vi "DI DAQ.vi"(11 "Queue ref":T1) -> ()   [LabVIEW 2022 SP3]
uses:
  Controls/All Queue.ctl
  Controls/DAQ case.ctl
  Controls/UI Data.ctl
  Controls/All Loop Status.ctl
  <vilib>/DAQmx/read.llb/DAQmx Read (Digital 1D Wfm NChan NSamp).vi
  Create Task/DI Create Task.vi
  <vilib>/DAQmx/configure/timing.llb/DAQmx Timing (Sample Clock).vi
  <vilib>/DAQmx/configure/trigger.llb/DAQmx Start Trigger (Time).vi
  Sub VI's/Global 1.vi
  <vilib>/DAQmx/miscellaneous.llb/DAQmx Fill In Error Info.vi
panel:
  # "TC channel list"
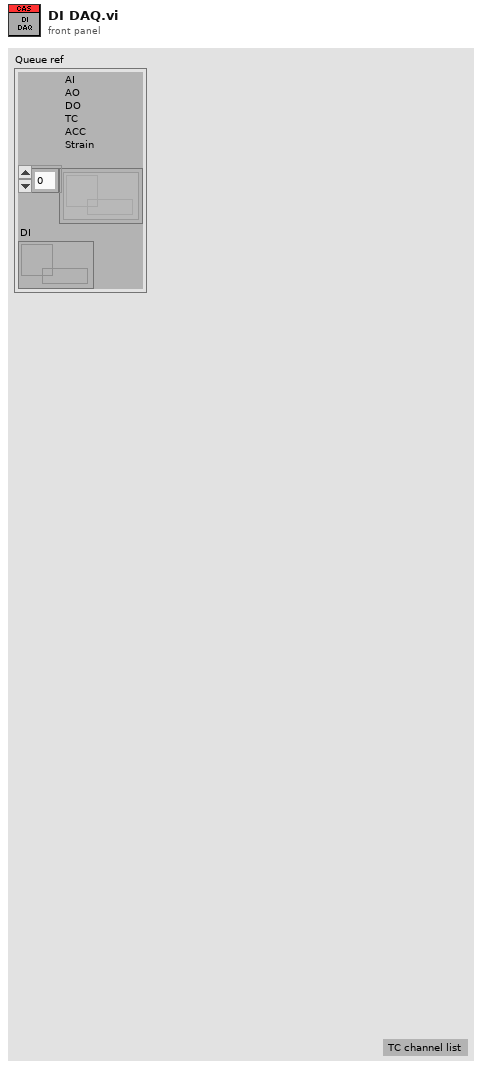
[diagram p1: front panel]
types:
  T1 = typedef "All Queue.ctl" = cluster{"AI\nAO\nDO\nTC\nACC\nStrain":refnum<queue>[], "DI":refnum<queue>}
  T2 = cluster{"in progress?":bool, "Queue ref":T1, "Start DAQ":refnum<notifier>, "UI Data":refnum<notifier>, "task out":refnum<k21>, "AI Ref":refnum<queue>, "SPC":i32}
  T3 = typedef "DAQ case.ctl" = enum16{"Initailise", "Create Task", "Polevent", "Acquire", "Stop DAQ", "Error", "Exit"}
  T4 = typedef "All Loop Status.ctl" = enum16{"AI", "AO", "DI", "DO", "TC", "Strain", "ACC", "RT", "Log"}
  T5 = enum16{"Init", "Read 'All'", "Read 'n'", "Read '1'", "Write '1'", "Write 'n'", "Write 'All'"}
  T6 = typedef "All Notifer.ctl" = cluster{"UI Data":refnum<notifier>, "Start DAQ":refnum<notifier>, "Start Log":refnum<notifier>}
  T7 = cluster{"Analog input":bool, "Analog Output":bool, "Digital input":bool, "Digital output":bool, "Thermocouple":bool, "Strain Gauge":bool, "Accelerometer":bool}
  T8 = typedef "Config.ctl" = cluster{"AO config":cluster{"Channel_Name":string, "Channel_Number":string, "Default_Value":dbl, "Units":string}[], "AI config":cluster{"Channel_Name":string, "Channel_Number":string, "Pre_Scale_min":dbl, "Pre_Scale_max":dbl, "Sensor_min":dbl, "Sensor_max":dbl, "Units":string}[], "DI config":cluster{"Channel_Name":string, "Channel_Number":string, "Default_Value":bool, "DI invert?":bool}[], "DO config":cluster{"Channel_Name":string, "Channel_Number":string, "Default_Value":bool, "DO invert?":bool}[], "TC config":cluster{"Channel_Name":string, "Channel_Number":string, "Pre_Scale_min":dbl, "Pre_Scale_max":dbl, "units":i32, " type":i32}[], "ACC config":cluster{"Channel_Name":string, "Channel_Number":string, "Pre_Scale_min":dbl, "Pre_Scale_max":dbl, "Terminal configuration":i32, "Sensitivity":dbl, "Sensitivity units":i32}[], "SG config":cluster{"Channel_Name":string, "Channel_Number":string, "Pre_Scale_min":dbl, "Pre_Scale_max":dbl}[], "Strain Gauge Settings":cluster{"poisson ratio":dbl, "nominal gage resistance":dbl, "gage factor":dbl}, "bridge information":cluster{"strain configuration":i32, "lead wire resistance":dbl, "initial bridge voltage":dbl, "voltage excitation source":i32, "voltage excitation value":dbl}, "Sample Rate":cluster{"AI Sample Rate":dbl, "AO Sample Rate":dbl, "DI Sample Rate":dbl, "TC Sample Rate":dbl, "DO Sample Rate":dbl, "SG Sample Rate":dbl, "ACC Sample Rate":dbl}}
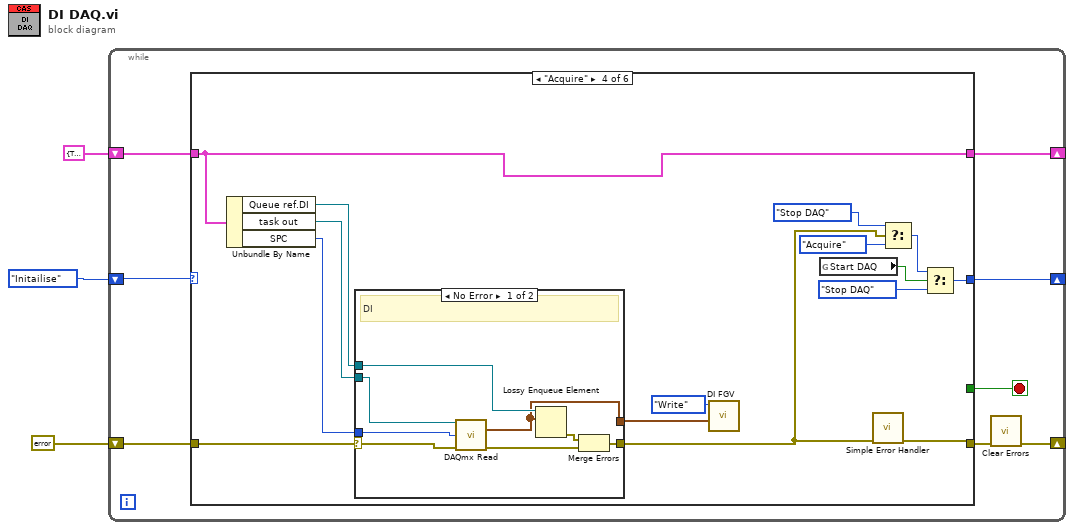
[diagram p0: block diagram]
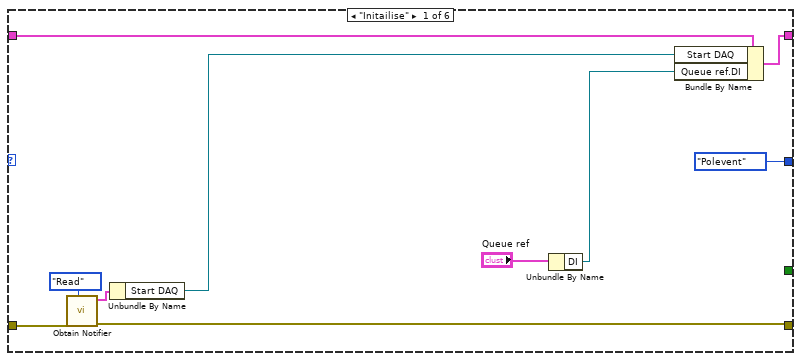
[diagram p2: hidden frame]
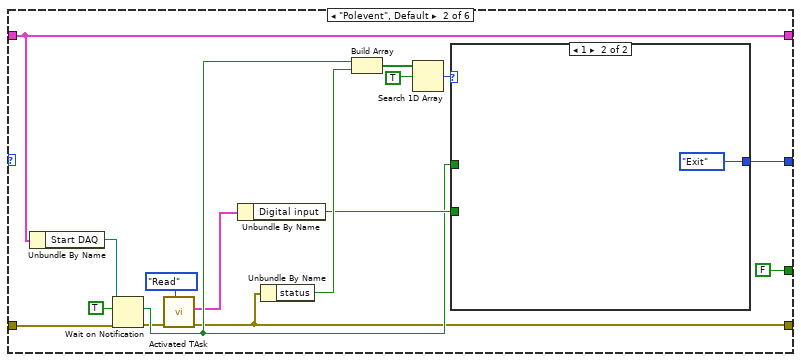
[diagram p3: hidden frame]
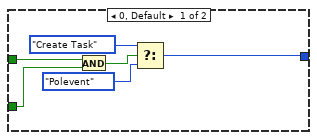
[diagram p4: hidden frame]
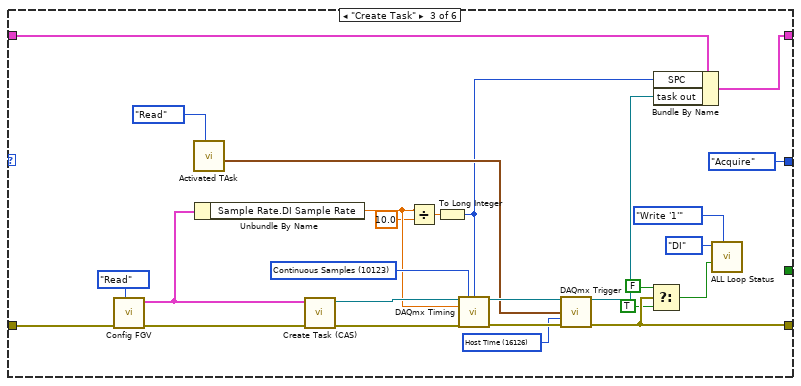
[diagram p5: hidden frame]
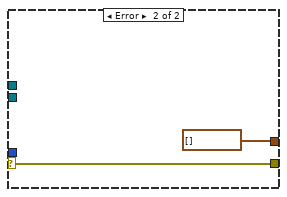
[diagram p6: hidden frame]
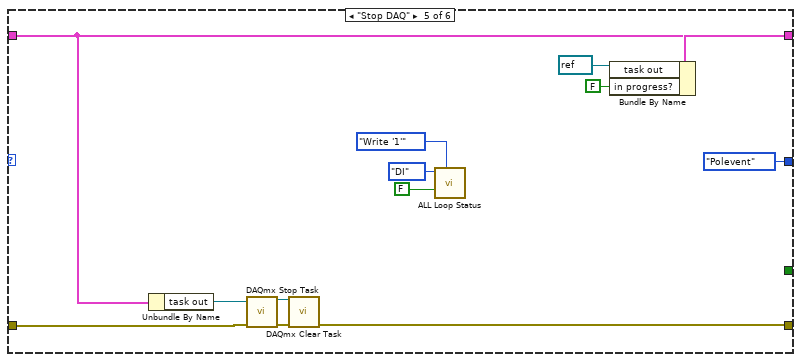
[diagram p7: hidden frame]
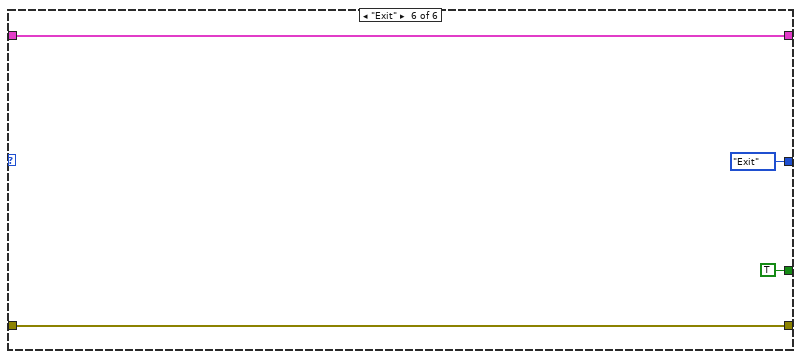
[diagram p8: hidden frame]
diagram:
  n1 = while {
    shift-right: [w4] -> _
    shift-left: errorcluster {"status"=FALSE, "code"=0, "source"=""} ("error out") -> [w10]
    shift-right: [w8] -> _
    shift-left: T2 {"in progress?"=TRUE, "Queue ref"={"AI\nAO\nDO\nTC\nACC\nStrain"=[], "DI"=refnum}, "Start DAQ"=refnum, "UI Data"=refnum, "task out"="", "AI Ref"=refnum, "SPC"=0} -> [w9]
    shift-right: [w7] -> _
    shift-left: DAQ_case."Initailise" -> [w6]
    stop <- w11 stop-if-true
    n2 = case shown="\"Acquire\"" w6 {
      tunnel: [_ FALSE _ _ _ TRUE] -> w11
      tunnel: w10 -> [w20 w25 w67 w78 w100 w112]
      tunnel: [w19 w23 w52 w72 w101 w112] -> w5
      tunnel: w9 -> [w17 w35 w69 w79 w105 w111]
      tunnel: [w15 w35 w68 w79 w106 w111] -> w8
      tunnel: [DAQ_case."Polevent" w36 DAQ_case."Acquire" w80 DAQ_case."Polevent" DAQ_case."Exit"] -> w7
      frame "Initailise" {
        n3 = call "Obtain Notifier.vi"("Case"=enum16{"Obtain", "Read"}."Read", "error in (no error)"=w20) -> ("error out"=w19:errorcluster, "notifiers out"=w18:T6)  [unwired: 8 in]
        n4 = Unbundle By Name(w18) -> ("Start DAQ"=w16:refnum<notifier>)
        n5 = Unbundle By Name("Queue ref") -> ("DI"=w12:refnum<queue>)
        n6 = Bundle By Name(cluster=w17, "Start DAQ"=w16, "Queue ref.DI"=w12) -> (w15:T2)
      }
      frame "Polevent", Default {
        n7 = Unbundle By Name(w35) -> ("Start DAQ"=w34:refnum<notifier>)
        n8 = Wait on Notification(notifier=w34, ignore previous (F)=TRUE, error in (no error)=w25) -> (notification=w26:bool, error out=w24:errorcluster)  [unwired: 1 in, 2 out]
        n9 = call "Activated TAsk.vi"("Enum"=enum16{"Read", "Write"}."Read", "error in (no error)"=w24) -> ("error out"=w23:errorcluster, "Activate Task 2"=w22:T7)  [unwired: 7 in, 1 out]
        n10 = Unbundle By Name(w22) -> ("Digital input"=w27:bool)
        n11 = Unbundle By Name(w23) -> ("status"=w33:bool)
        n12 = Build Array(w26, w33) -> (w31:bool[])
        n13 = Search 1D Array(1D array=w31, element=TRUE) -> (index of element=w29:i32)  [unwired: 1 in]
        n14 = case shown="1" w29 {
          tunnel: [w42 DAQ_case."Exit"] -> w36
          tunnel: w27 -> [w39 _]
          tunnel: w26 -> [w38 _]
          frame 0, Default {
            n15 = And(x=w38, y=w39) -> (x .and. y?=w40:bool)
            n16 = Select(t=DAQ_case."Create Task", s=w40, f=DAQ_case."Polevent") -> (s? t:f=w42:T3)
          }
          frame 1 {
          }
        }
      }
      frame "Create Task" {
        w57 = 16126 items=["Host Time"=16126, "I/O Device Time"=16127] ("timescale")
        w59 = 10123 items=["Finite Samples"=10178, "Continuous Samples"=10123, "Hardware Timed Single Point"=12522] ("sample mode")
        n17 = call "Config FGV.vi"("Enum"=enum16{"Read", "Write"}."Read", "error in (no error)"=w67) -> ("error out"=w64:errorcluster, "Data"=w49:T8)  [unwired: 8 in]
        n18 = call "Activated TAsk.vi"("Enum"=enum16{"Read", "Write"}."Read") -> ("Start Time"=w58:timestamp)  [unwired: 8 in, 2 out]
        n19 = Unbundle By Name(w49) -> ("Sample Rate.DI Sample Rate"=w48:dbl)
        n20 = call-poly "Create Task (CAS).vi"("error in"=w64, "Config"=w49) -> ("error out"=w61:errorcluster, "DI Task"=w63:refnum<k21>)  [unwired: 7 in, 1 out]
        n21 = Divide(x=w48, y=10.0) -> (x/y=w46:dbl)
        n22 = To Long Integer(number=w46) -> (32bit integer=w45:i32)
        n23 = call-poly <vilib>:"DAQmx Timing.vi"("task/channels in"=w63, "sample mode"=w59, "samples per channel"=w45, "rate"=w48, "error in"=w61) -> ("task out"=w62:refnum<k21>, "error out"=w60:errorcluster)  [unwired: 9 in]
        n24 = call-poly <vilib>:"DAQmx Trigger.vi"("task/channels in"=w62, "when"=w58, "timescale"=w57, "error in"=w60) -> ("task out"=w56:refnum<k21>, "error out"=w52:errorcluster)  [unwired: 10 in]
        n25 = Select(t=FALSE, s=w52, f=TRUE) -> (s? t:f=w53:bool)
        n26 = Bundle By Name(cluster=w69, "SPC"=w45, "task out"=w56) -> (w68:T2)
        n27 = call "ALL Loop Status.vi"("Option"=T5."Write '1'", "Status"=w53, "Loop"=All_Loop_Status."DI") -> ()  [unwired: 6 in, 3 out]
      }
      frame "Acquire" {
        n28 = Unbundle By Name(w79) -> ("Queue ref.DI"=w77:refnum<queue>, "task out"=w76:refnum<k21>, "SPC"=w71:i32)
        n29 = case shown="No Error" w78 {
          selector: w78 -> [w89 w95]
          tunnel: w76 -> [w88 _]
          tunnel: [w91 w95] -> w73
          tunnel: w77 -> [w90 _]
          tunnel: [w87 digitalwaveform[] [] ("data")] -> w74
          tunnel: w71 -> [w86 _]
          frame No Error {
            # "DI"
            n30 = call-poly <vilib>:"DAQmx Read.vi"("task/channels in"=w88, "number of samples per channel"=w86, "error in"=w89) -> ("data"=w87:digitalwaveform[], "error out"=w92:errorcluster)  [unwired: 10 in, 1 out]
            n31 = Lossy Enqueue Element(queue=w90, element=w87) -> (error out=w93:errorcluster)  [unwired: 1 in, 3 out]
            n32 = Merge Errors(w93, w92) -> (w91:errorcluster)
          }
          frame Error {
          }
        }
        n33 = call "DI FGV.vi"("DI Data"=w74, "Enum"=enum16{"Read", "Write"}."Write") -> ()  [unwired: 9 in, 1 out]
        n34 = global read "Global 1.vi" "Start DAQ"() -> (w83:bool)
        n35 = call <vilib>:"Simple Error Handler.vi"("error in (no error)"=w73) -> ("error out"=w72:errorcluster)  [unwired: 4 in, 4 out]
        n36 = Select(t=DAQ_case."Stop DAQ", s=w73, f=DAQ_case."Acquire") -> (s? t:f=w82:T3)
        n37 = Select(t=w82, s=w83, f=DAQ_case."Stop DAQ") -> (s? t:f=w80:T3)
      }
      frame "Stop DAQ" {
        n38 = Unbundle By Name(w105) -> ("task out"=w99:refnum<k21>)
        n39 = call <vilib>:"DAQmx Stop Task.vi"("task/channels in"=w99, "error in"=w100) -> ("task out"=w98:refnum<k21>, "error out"=w102:errorcluster)  [unwired: 12 in]
        n40 = call <vilib>:"DAQmx Clear Task.vi"("task in"=w98, "error in"=w102) -> ("error out"=w101:errorcluster)  [unwired: 13 in]
        n41 = call "ALL Loop Status.vi"("Option"=T5."Write '1'", "Status"=FALSE, "Loop"=All_Loop_Status."DI") -> ()  [unwired: 6 in, 3 out]
        n42 = Bundle By Name(cluster=w105, "task out"=refnum<k21> refnum, "in progress?"=FALSE) -> (w106:T2)
      }
      frame "Exit" {
      }
    }
    n43 = call <vilib>:"Clear Errors.vi"("error in (no error)"=w5) -> ("error out"=w4:errorcluster)  [unwired: 5 in, 1 out]
  }
